vi "SECS Bridge Log View.vi"() -> ()   [LabVIEW 2020, in "SECS Bridge.lvlib"]
uses:
  SECS Bridge.lvlib
  SubVI/File FGV Method.ctl
  PPL/Universal Function.lvlibp
panel:
  in  "Stop":bool
  in  "Export":bool
  in  "Notifier Data":i32(listbox)
  in  "Log File":string(combo)
  in  "Load":bool
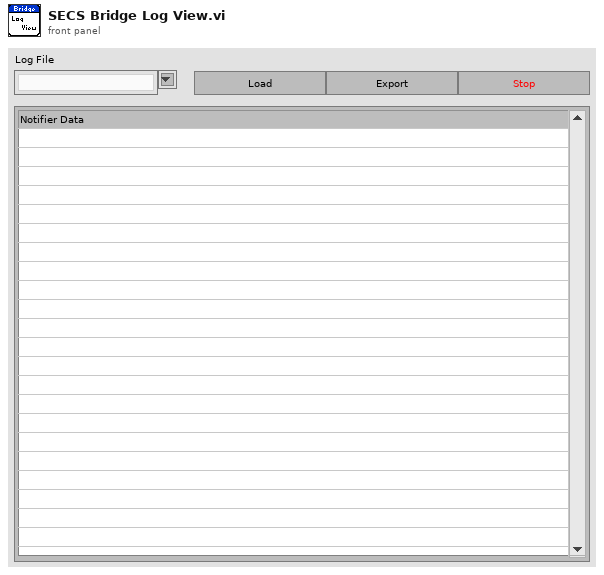
[diagram p1: front panel]
types:
  T1 = typedef "SECS Bridge.lvlib/File FGV Method.ctl" = enum16{"Get", "Put", "Read", "Write"}
  T2 = typedef "SECS Bridge.lvlib/Configuration.ctl" = cluster{"T3(Reply Timeout)":i32, "T5(Separation Timeout)":i32, "T6(Control Timeout)":i32, "T7(Not Selected Timeout)":i32, "T8(Inter-Character Timeout)":i32, "Session ID":u16, "Log Path":path, "IP Address":string, "Port":u16}
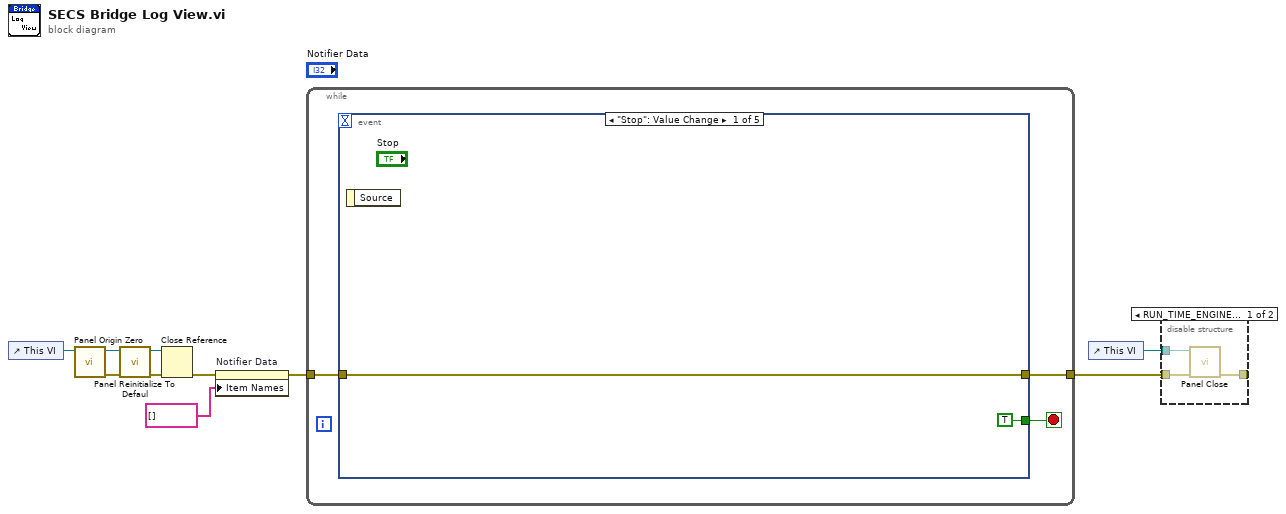
[diagram p0: block diagram]
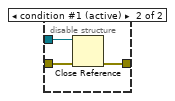
[diagram p2: hidden frame]
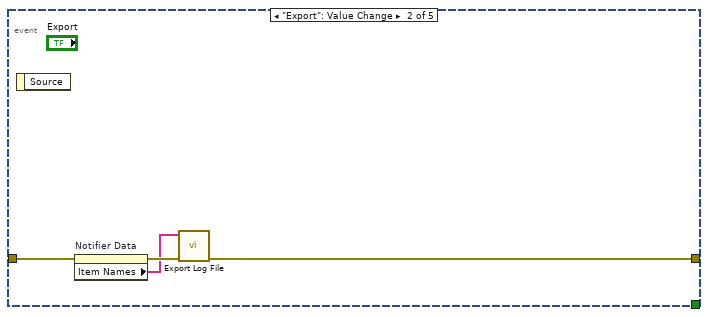
[diagram p3: hidden frame]
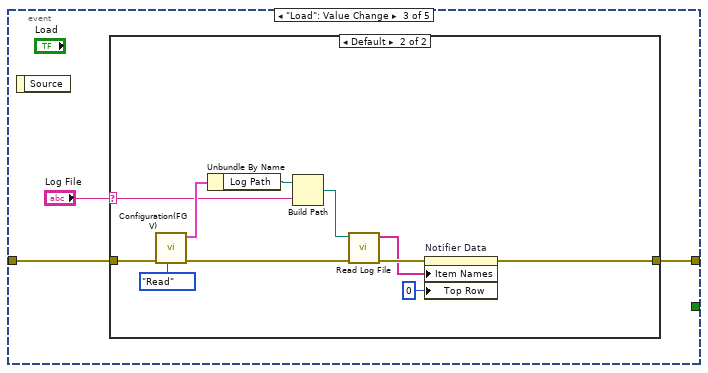
[diagram p4: hidden frame]
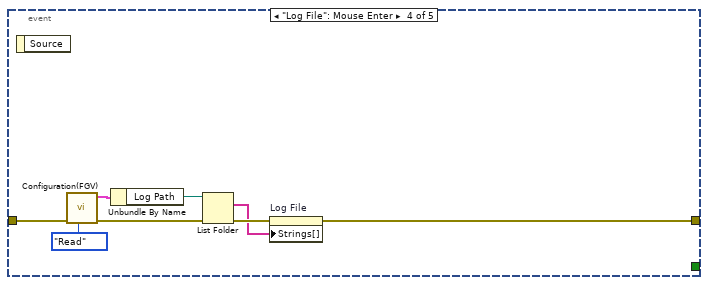
[diagram p6: hidden frame]
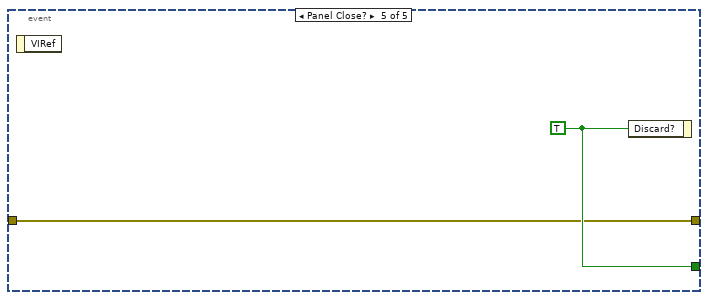
[diagram p7: hidden frame]
diagram:
  n1 = control-ref of="This VI"() -> (w10:refnum<vi>)
  n2 = call "Panel Origin Zero.vi"("VI Refnum In"=w10) -> ("error out"=w8:errorcluster, "VI Refnum Out"=w9:refnum<vi>)  [unwired: 9 in]
  n3 = call "Panel Reinitialize To Defaul.vi"("error in"=w8, "VI Refnum In"=w9) -> ("error out"=w7:errorcluster, "VI Refnum Out"=w6:refnum<vi>)  [unwired: 8 in]
  n4 = Close Reference(reference=w6, error in (no error)=w7) -> (error out=w3:errorcluster)
  n5 = property on="Notifier Data" class="LstBox (strict)"(error in=w3, "Item Names"=string[] []) -> (error out=w2:errorcluster)  [unwired: 1 in, 1 out]
  n6 = while {
    tunnel: [w13] -> w5
    tunnel: w2 -> [w11]
    stop <- w12 stop-if-true
    n7 = event shown="[0] \"Stop\": Value Change" {
      selector: _ -> [_ _ _ _ _]
      dyn-events: _ -> [_ _ _ _ _]
      timeout: _ -> [_ _ _ _ _]
      tunnel: [w15 w16 w22 w35 w43] -> w13
      tunnel: [TRUE ("Discard?") _ _ _ w44] -> w12
      tunnel: w11 -> [w15 w19 w21 w36 w43]
      event "Stop": Value Change {
        n8 = event-data() -> ()  [unwired: 1 in, 1 out]
      }
      event "Export": Value Change {
        n9 = event-data() -> ()  [unwired: 1 in, 1 out]
        n10 = property on="Notifier Data" class="LstBox (strict)"(error in=w19) -> (error out=w18:errorcluster, "Item Names"=w17:string[])  [unwired: 1 in, 1 out]
        n11 = call "Export Log File.vi"("error in"=w18, "File Data"=w17) -> ("error out"=w16:errorcluster)  [unwired: 9 in]
      }
      event "Load": Value Change {
        n12 = event-data() -> ()  [unwired: 1 in, 1 out]
        n13 = case shown="Default" "Log File" {
          selector: "Log File" -> [_ w28]
          tunnel: [w23 w25] -> w22
          tunnel: w21 -> [w23 w29]
          frame "" {
          }
          frame Default {
            n14 = call "Configuration(FGV).vi"("File FGV Method"=File_FGV_Method."Read", "error in"=w29) -> ("error out"=w31:errorcluster, "Configuration Out"=w34:T2)  [unwired: 8 in]
            n15 = Unbundle By Name(w34) -> ("Log Path"=w32:path)
            n16 = Build Path(base path=w32, name or relative path=w28) -> (appended path=w30:path)
            n17 = call "Read Log File.vi"("error in"=w31, "Path"=w30) -> ("error out"=w27:errorcluster, "File Data"=w26:string[])  [unwired: 8 in]
            n18 = property on="Notifier Data" class="LstBox (strict)"(error in=w27, "Item Names"=w26, "Top Row"=0) -> (error out=w25:errorcluster)  [unwired: 1 in, 1 out]
          }
        }
      }
      event "Log File": Mouse Enter {
        n19 = event-data() -> ()  [unwired: 1 in, 1 out]
        n20 = call "Configuration(FGV).vi"("File FGV Method"=File_FGV_Method."Read", "error in"=w36) -> ("error out"=w41:errorcluster, "Configuration Out"=w40:T2)  [unwired: 8 in]
        n21 = Unbundle By Name(w40) -> ("Log Path"=w42:path)
        n22 = List Folder(path=w42, error in=w41) -> (filenames=w37:string[], error out=w38:errorcluster)  [unwired: 2 in, 2 out]
        n23 = property on="Log File" class="CmbBox"(error in=w38, "Strings[]"=w37) -> (error out=w35:errorcluster)  [unwired: 1 in, 1 out]
      }
      event Panel Close? {
        w44 = TRUE ("Discard?")
        n24 = event-data() -> ()  [unwired: 1 in, 1 out]
        n25 = event-data("Discard?"=w44) -> ()  [unwired: 1 in, 1 out]
      }
    }
  }
  n26 = control-ref of="This VI"() -> (w4:refnum<vi>)
  n27 = disable-structure shown="RUN_TIME_ENGINE==True, Default" {
    disable-tunnel: w5 -> [w47 w50]
    disable-tunnel: w4 -> [w46 w48]
    disable-tunnel: [w45 w49] -> _
    frame condition #0 {
      n28 = call "Panel Close.vi"("error in"=w47, "VI Refnum"=w46) -> ("error out"=w45:errorcluster)  [unwired: 9 in]
    }
    frame condition #1 (active) {
      n29 = Close Reference(reference=w48, error in (no error)=w50) -> (error out=w49:errorcluster)
    }
  }
